vi "Send ABORT.vi"(8 "error in (no error)":errorcluster, 9 "Abort Request":T1, 11 "WAMP Client in":refnum<class "WAMP Client.lvclass">) -> (0 "error out":errorcluster, 3 "WAMP Client out":refnum<class "WAMP Client.lvclass">)   [LabVIEW 2020, in "wamplv.lvlib" / "WAMP Client.lvclass"]
uses:
  WAMP Client.lvclass
  TypeDef/Termination Reason.ctl
  TypeDef/Termination Reason Enum.ctl
  WAMP Client.lvclass/WAMP Client.ctl
  Comm Handlers/ICommHandler/ICommHandler.lvclass
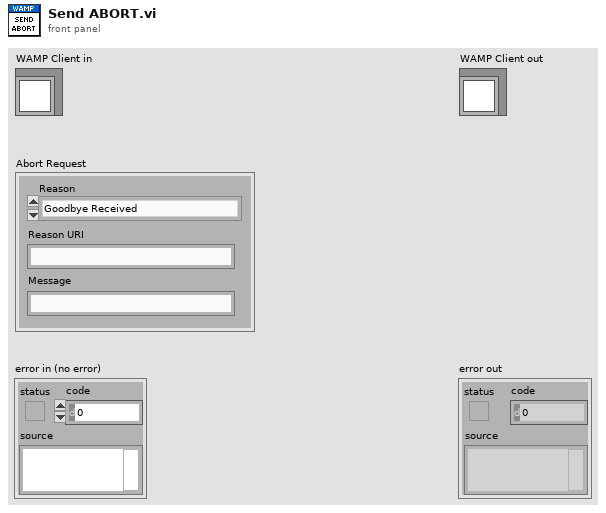
[diagram p1: front panel]
types:
  T1 = typedef "wamplv.lvlib/WAMP Client.lvclass/Termination Reason.ctl" = cluster{"Reason":T2, "Reason URI":string, "Message":string}
  T2 = typedef "wamplv.lvlib/WAMP Client.lvclass/Termination Reason Enum.ctl" = enum16{"Goodbye Received", "Abort Received", "Send Goodbye", "Send Abort", "Read Loop Failure", "Write Loop Failure", "Message Loop Failure"}
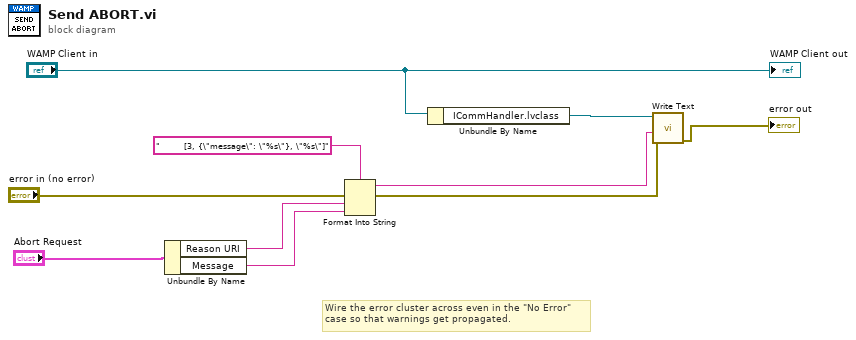
[diagram p0: block diagram]
diagram:
  # "Wire the error cluster across even in the \"No Error\"\ncase so that warnings get propagated."
  n1 = Unbundle By Name("Abort Request") -> ("Reason URI"=w6:string, "Message"=w5:string)
  n2 = Format Into String(format string="        [3, {\"message\": \"%s\"}, \"%s\"]", error in="error in (no error)", w6, w5) -> (resulting string=w3:string, error out=w2:errorcluster)  [unwired: 1 in]
  n3 = Unbundle By Name("WAMP Client in") -> ("ICommHandler.lvclass"=w7:refnum<class "ICommHandler.lvclass">)
  n4 = call-dynamic "Write Text.vi"("error in (no error)"=w2, "String"=w3, "ICommHandler in"=w7) -> ("error out"=→"error out":errorcluster)  [unwired: 7 in, 1 out]
  "WAMP Client out" <- "WAMP Client in"
